vi "Lesson 1, Locating Controls, Functions & VIs.vi"() -> ()   [LabVIEW 2022 SP3]
uses:
  <vilib>/Analysis/Matrix/Datatypes/RealMatrix.ctl
  <vilib>/Analysis/Matrix/NI_Matrix.lvlib
panel:
  in  "Real Matrix":T1
  in  "Slide":dbl(slide) scale=0.0..10.0
  in  "Numeric":dbl
  out "Message":string
  out "Warning":bool
  in  "Seconds":dbl
  in  "Minutes":dbl
  in  "Hours":dbl
  in  "Total Time in Seconds":dbl
  in  "String":string
  out "Output":dbl
  in  "B":dbl
  in  "A":dbl
  # "VI to Add Two Numbers Together (Intoduction to LabCore)"
  # "Locating Controls, Functions & VIs"
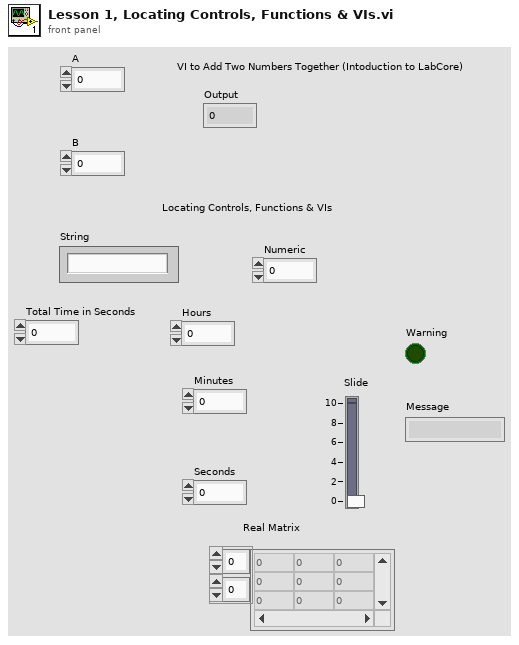
[diagram p1: front panel]
types:
  T1 = typedef "NI_Matrix.lvlib/RealMatrix.ctl" = dbl[][]
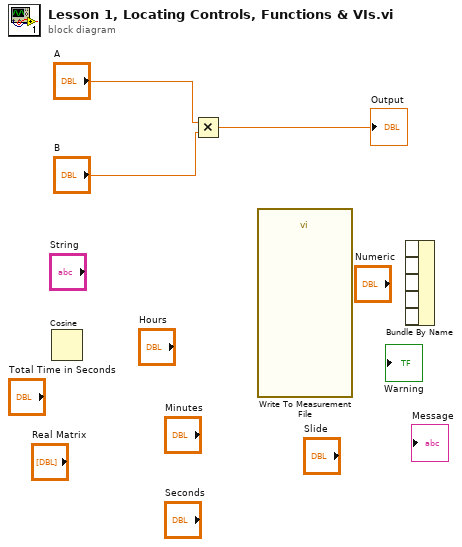
[diagram p0: block diagram]
diagram:
  n1 = Cosine() -> ()  [unwired: 1 in, 1 out]
  n2 = Multiply(x="A", y="B") -> (x*y=→"Output":dbl)
  n3 = call "Write To Measurement File"() -> ()  [unwired: 17 in, 3 out]
  n4 = Bundle By Name() -> ()  [unwired: 6 in, 1 out]
